vi "Write Job Description.vi"(8 "error in (no error)":errorcluster, 10 "Job Description":string, 11 "Build Job in":refnum<class "Build Job.lvclass">) -> (0 "error out":errorcluster, 3 "Build Job out":refnum<class "Build Job.lvclass">)   [LabVIEW 2014, in "Build Job.lvclass"]
uses:
  Build Job.lvclass
  Build Job.lvclass/Build Job.ctl
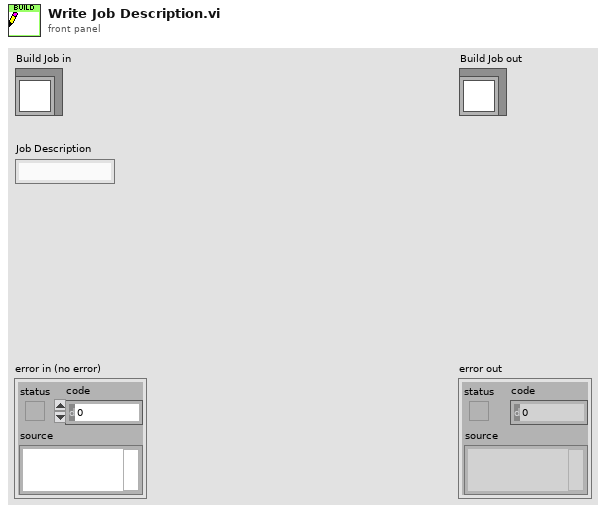
[diagram p1: front panel]
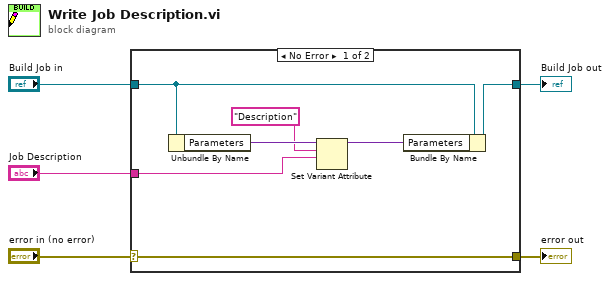
[diagram p0: block diagram]
diagram:
  n1 = case shown="No Error" "error in (no error)" {
    selector: "error in (no error)" -> [w12 w13]
    tunnel: [w12 w13] -> w4
    tunnel: [w11 w14] -> w2
    tunnel: "Build Job in" -> [w10 w14]
    tunnel: "Job Description" -> [w6 _]
    frame No Error {
      n2 = Unbundle By Name(w10) -> ("Parameters"=w9:variant)
      n3 = Set Variant Attribute(Variant=w9, name="Description", value=w6) -> (Variant out=w8:variant)  [unwired: 1 in, 2 out]
      n4 = Bundle By Name(cluster=w10, "Parameters"=w8) -> (w11:refnum<class "Build Job.lvclass">)
    }
    frame Error {
    }
  }
  "error out" <- w4
  "Build Job out" <- w2
